vi "ueye grab image.vi"(8 "error in (no error)":errorcluster, 10 "Image In":T1, 11 "Camera in":refnum<k24>) -> (0 "error out":errorcluster, 2 "Image Out":T1, 3 "Camera out":refnum<k24>)   [LabVIEW 2024, in "Vision.lvlib"]
uses:
  Vision.lvlib
  <vilib>/vision/Image Controls.llb/IMAQ Image.ctl
  C:/Users/cfang/Desktop/nebraska-silicon-lab/pixel-gantry-control/Gantry/Shared Components/bin.bak/uEyeDotNet.dll
  bin.bak/uEyeDotNet.dll
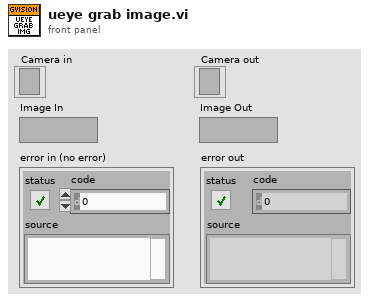
[diagram p1: front panel]
types:
  T1 = typedef "IMAQ Image.ctl" = refnum<image>
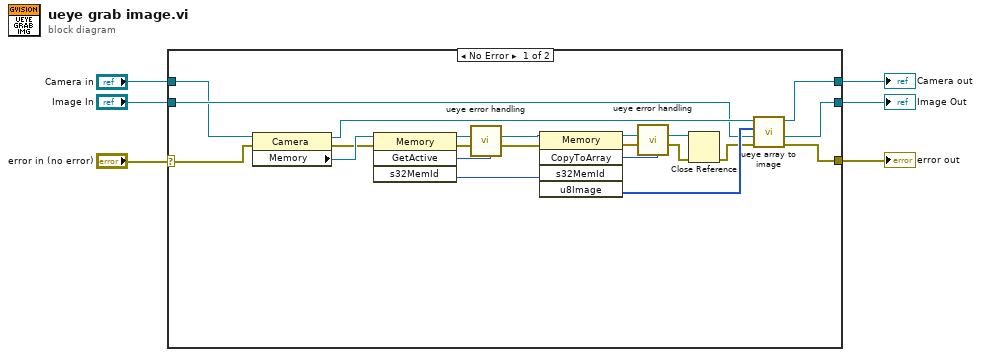
[diagram p0: block diagram]
diagram:
  n1 = case shown="No Error" "error in (no error)" {
    selector: "error in (no error)" -> [w7 w27]
    tunnel: [w12 w27] -> w6
    tunnel: "Image In" -> [w11 w29]
    tunnel: [w10 w29] -> w4
    tunnel: [w9 w28] -> w3
    tunnel: "Camera in" -> [w8 w28]
    frame No Error {
      n2 = property class="Camera"(reference=w8, error in=w7) -> (reference out=w23:refnum<k24>, error out=w25:errorcluster, "Memory"=w26:refnum<k24>)
      n3 = invoke class="Memory" method="GetActive"(reference=w26, error in=w25) -> (reference out=w18:refnum<k24>, error out=w21:errorcluster, "GetActive"=w20:i32, "s32MemId"=w24:i32)  [unwired: 2 in]
      n4 = call "ueye error handling.vi"("Error Code"=w20, "reference in"=w18, "Error In"=w21) -> ("Error Out"=w19:errorcluster)  [unwired: 8 in]
      n5 = invoke class="Memory" method="CopyToArray"(reference=w18, error in=w19, "s32MemId"=w24) -> (reference out=w15:refnum<k24>, error out=w17:errorcluster, "CopyToArray"=w16:i32, "u8Image"=w22:u8[])  [unwired: 2 in, 1 out]
      n6 = call "ueye error handling.vi"("Error Code"=w16, "reference in"=w15, "Error In"=w17) -> ("Error Out"=w14:errorcluster)  [unwired: 8 in]
      n7 = Close Reference(reference=w15, error in (no error)=w14) -> (error out=w13:errorcluster)
      n8 = call "ueye array to image.vi"("Error In"=w13, "Image In"=w11, "InArray"=w22, "Camera Reference"=w23) -> ("Error Out"=w12:errorcluster, "Image Out"=w10:T1, "Camera reference out"=w9:refnum<k24>)  [unwired: 5 in]
    }
    frame Error {
    }
  }
  "error out" <- w6
  "Image Out" <- w4
  "Camera out" <- w3
